vi "beginPrepareTriplePassPlay.vi"(8 "error in (no error)":errorcluster, 9 "Game":refnum<class "Game.lvclass">, 10 "last command_interpreted":T1, 11 "PrepareTriplePassPlay in":refnum<class "PrepareTriplePassPlay.lvclass">) -> (0 "error out":errorcluster, 2 "Boolean":bool, 3 "PrepareTriplePassPlay out":refnum<class "PrepareTriplePassPlay.lvclass">)   [LabVIEW 2023, in "PrepareTriplePassPlay.lvclass"]
uses:
  PrepareTriplePassPlay.lvclass
  Game_class/Game.lvclass
  Referee_class/command_interpreted.ctl
  Game_class/Game.lvclass/Game.ctl
  Referee_class/Referee.lvclass/Referee.ctl
  Parameters_class/Parameters.lvclass/Parameters.ctl
  Game_class/Read Referee.vi
  Game_class/Read Parameters.lvclass.vi
  Game_class/Read BallRef.vi
  Game_class/Read Utilities.lvclass.vi
  Game_class/Read FieldRef.vi
  Parameters_class/Read RollToPass.vi
  Referee_class/Read command_interpreted.vi
  Referee_class/Referee.lvclass
  Parameters_class/Parameters.lvclass
  Ball_class/Ball.lvclass
  Utilities_class/Utilities.lvclass
  Field_class/Field.lvclass
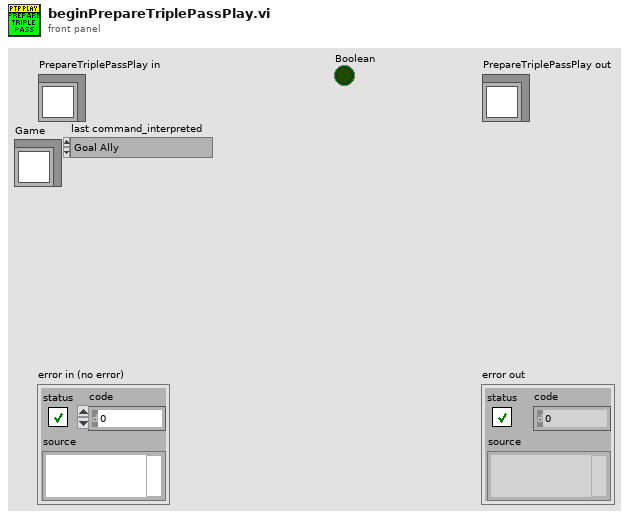
[diagram p1: front panel]
types:
  T1 = typedef "command_interpreted.ctl" = enum16{"Goal Ally", "Goal Enemy", "Ball Placement Enemy", "Ball Placement Ally", "Normal Half Time", "Extra Time  Break", "Extra Half Time", "None", "Post Game", "PKA Normal Start", "Prepare Kickoff Ally", "PKE Normal Start", "Prepare Kickoff Enemy", "Force Start", "Halt", "Timeout", "Prepare Penalty Ally", "Prepare Penalty Enemy", "PPA NormalStart", "PPE Normal Start", "Indirect Free Ally", "Direct Free Enemy", "Direct Free Ally", "Indirect Free Enemy", "Stop"}
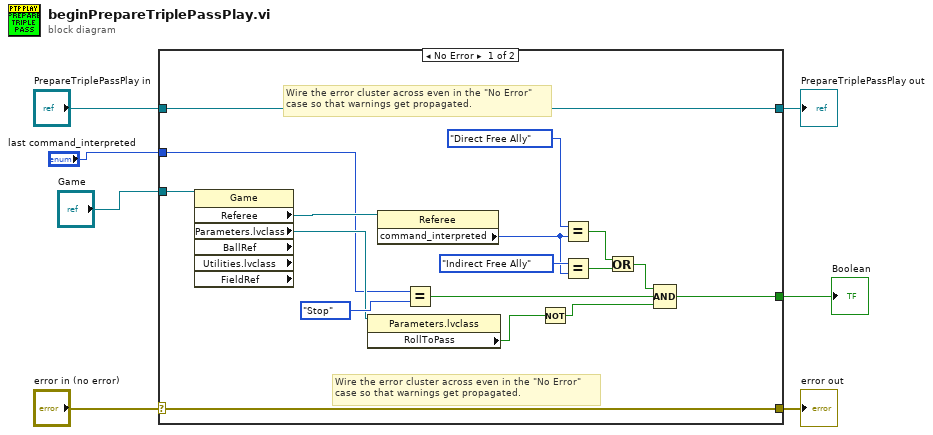
[diagram p0: block diagram]
diagram:
  n1 = case shown="No Error" "error in (no error)" {
    selector: "error in (no error)" -> [w23 w26]
    tunnel: [w23 w26] -> w6
    tunnel: [w24 w25] -> w4
    tunnel: "PrepareTriplePassPlay in" -> [w24 w25]
    tunnel: "Game" -> [w10 _]
    tunnel: "last command_interpreted" -> [w9 _]
    tunnel: [w8 _] -> w1
    frame No Error {
      # "Wire the error cluster across even in the \"No Error\"\ncase so that warnings get propagated."
      # "Wire the error cluster across even in the \"No Error\"\ncase so that warnings get propagated."
      n2 = property class="Game" props=["Referee", "Parameters.lvclass", "BallRef", "Utilities.lvclass", "FieldRef"](reference=w10) -> ("Referee"=w22:refnum<class "Referee.lvclass">, "Parameters.lvclass"=w13:refnum<class "Parameters.lvclass">)  [unwired: 1 in, 5 out]
      n3 = property class="Parameters.lvclass"(reference=w13) -> ("RollToPass"=w12:bool)  [unwired: 1 in, 2 out]
      n4 = property class="Referee"(reference=w22) -> ("command_interpreted"=w18:T1)  [unwired: 1 in, 2 out]
      n5 = Equal?(x=w9, y=command_interpreted."Stop" ("command_interpreted")) -> (x = y?=w14:bool)
      n6 = Not(x=w12) -> (.not. x?=w11:bool)
      n7 = Equal?(x=command_interpreted."Direct Free Ally" ("command_interpreted"), y=w18) -> (x = y?=w17:bool)
      n8 = Equal?(x=command_interpreted."Indirect Free Ally" ("command_interpreted"), y=w18) -> (x = y?=w15:bool)
      n9 = Or(x=w17, y=w15) -> (x .or. y?=w16:bool)
      n10 = Compound Arithmetic op=AND(w16, w14, w11) -> (w8:bool)
    }
    frame Error {
    }
  }
  "error out" <- w6
  "PrepareTriplePassPlay out" <- w4
  "Boolean" <- w1
